vi "Load.vi"(8 "error in":errorcluster, 11 "Gantry In":refnum<class "Gantry Class.lvclass">) -> (0 "error out":errorcluster, 3 "Grabber Tool out":refnum<class "GrabberTool Class.lvclass">)   [LabVIEW 2011, in "GrabberTool Class.lvclass"]
uses:
  GrabberTool Class.lvclass
  Gantry Class/Gantry Class.lvclass
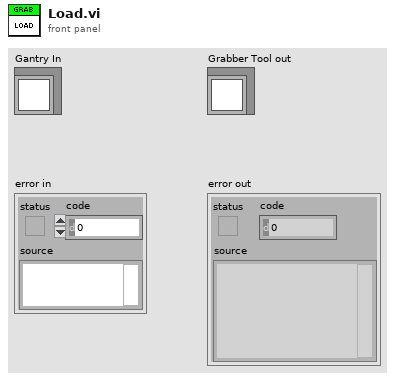
[diagram p1: front panel]
types:
  T1 = enum16{"None", "Grabber", "Picker", "Tool Setter"}
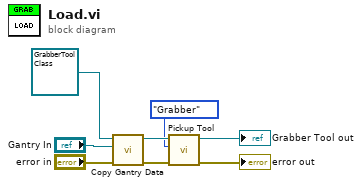
[diagram p0: block diagram]
diagram:
  n1 = call "Copy Gantry Data.vi"("error in"="error in", "Gantry Source"="Gantry In", "Gantry Dest"=refnum<class "GrabberTool Class.lvclass"> refnum ("CameraTool Class in")) -> ("error out"=w3:errorcluster, "Gantry Result"=w5:refnum<class "GrabberTool Class.lvclass">)  [unwired: 7 in]
  n2 = call-dynamic "Pickup Tool.vi"("error in"=w3, "Tool"=T1."Grabber", "Gantry in"=w5) -> ("error out"=→"error out":errorcluster, "Gantry out"=→"Grabber Tool out":refnum<class "GrabberTool Class.lvclass">)  [unwired: 7 in]
